vi "EnvelopDetector(SubVI).vi"(1 "modulated signal (time-domain)":waveform(dbl)) -> (0 "Demodulated DSB (time)":dynamicdata(graph) caption="Filtered Signal")   [LabVIEW 2010]
uses:
  <vilib>/ptbypt/NI_PtbyPt.lvlib
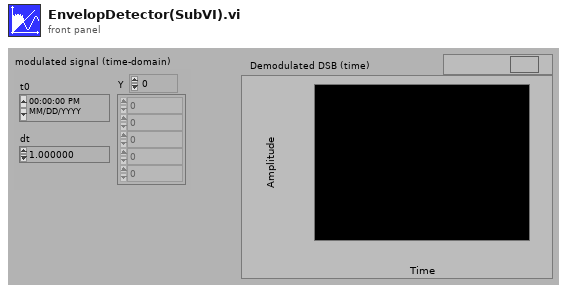
[diagram p1: front panel]
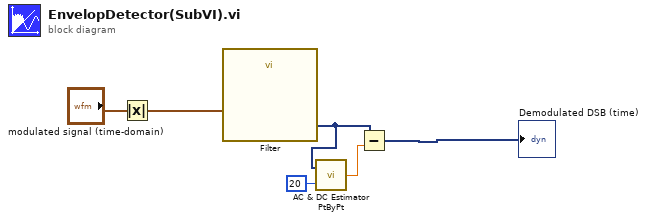
[diagram p0: block diagram]
diagram:
  n1 = Absolute Value(x="modulated signal (time-domain)") -> (abs(x)=w5:waveform(dbl))
  n2 = call "Filter"("Signal"=w5) -> ("Filtered Signal"=w2:dynamicdata)  [unwired: 9 in, 1 out]
  n3 = call <vilib>:"AC & DC Estimator PtByPt.vi"("signal"=w2, "sample length"=20) -> ("DC estimate (V)"=w3:dbl)  [unwired: 1 in, 2 out]
  n4 = Subtract(x=w2, y=w3) -> (x-y=→"Demodulated DSB (time)":dynamicdata)
